vi "get object tags.vi"(1 "can select all services":bool, 2 "Object":string, 5 "error in (no error)":errorcluster) -> (16 "services":string[](array[string]), 17 "descriptors":string[](array[string]), 19 "error out":errorcluster)   [LabVIEW 2014, in "PTUtils.lvlib"]
doc: "Gets the services published by an object by queying its DIM server."
uses:
  PTUtils.lvlib
  CSCore/CSSystem/CoreLib/CoreLib.lvlib
  CSlibraries/UtilityLib/UtilityLib.lvlib
  CSlibraries-extern/DimLVEvent/LVDimInterface/LVDimInterface.lvlib
  CSCore/CSSystem/CSSystemLib/CSSystemLib.lvlib
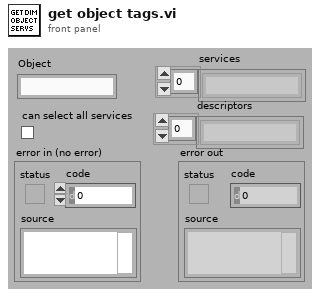
[diagram p1: front panel]
types:
  T1 = cluster{"string without white spaces":string, "string without white spaces":string}
  T2 = cluster{"string without white spaces":string, "string without white spaces":string}[]
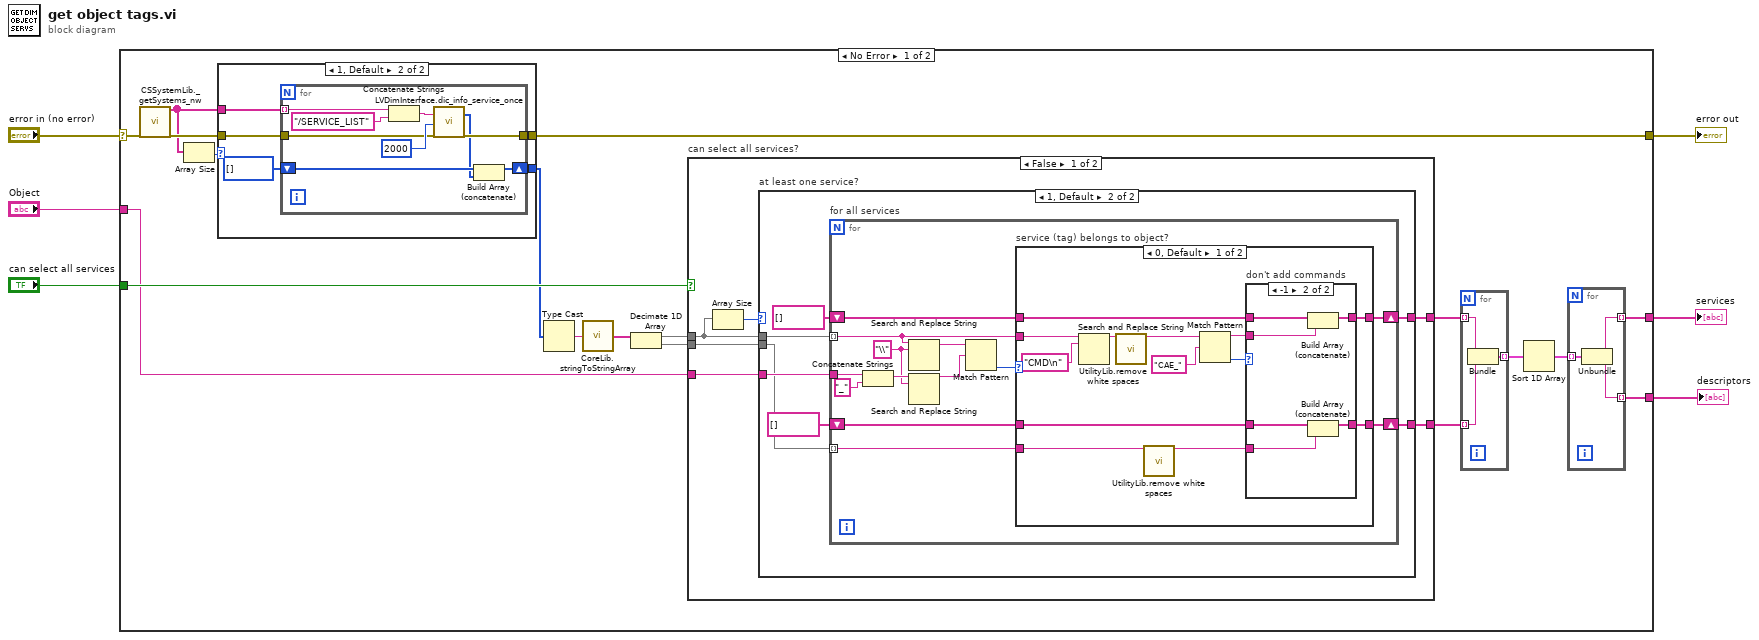
[diagram p0: block diagram]
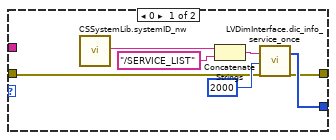
[diagram p2: hidden frame]
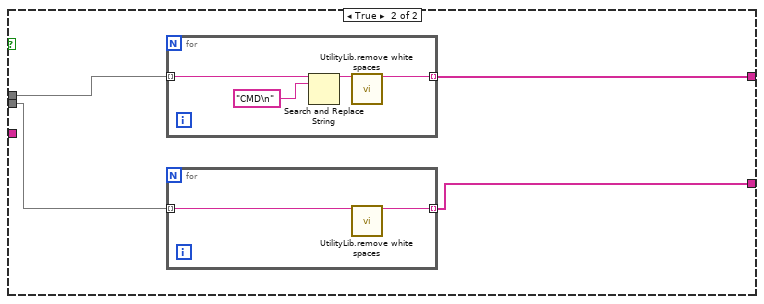
[diagram p6: hidden frame]
diagram:
  n1 = case shown="No Error" "error in (no error)" {
    selector: "error in (no error)" -> [w17 w111]
    tunnel: [w23 w111] -> w6
    tunnel: "can select all services" -> [w24 _]
    tunnel: "Object" -> [w14 _]
    tunnel: [w8 _] -> w2
    tunnel: [w7 _] -> w1
    frame No Error {
      n2 = call "CSSystemLib._getSystems_nw.vi"("error in (no error)"=w17) -> ("CSSystems"=w16:string[], "error out"=w18:errorcluster)  [unwired: 16 in, 1 out]
      n3 = Array Size(array=w16) -> (size(s)=w15:i32)
      n4 = case shown="1, Default" w15 {
        tunnel: [w32 w42] -> w23
        tunnel: [w34 w41] -> w22
        tunnel: w18 -> [w31 w39]
        tunnel: w16 -> [_ w38]
        frame 0 {
          n5 = call "CSSystemLib.systemID_nw.vi"() -> ("systemID out"=w33:string)  [unwired: 18 in, 1 out]
          n6 = Concatenate Strings(w33, "/SERVICE_LIST" ("string")) -> (w36:string)
          n7 = call "LVDimInterface.dic_info_service_once.vi"("serviceName"=w36, "timeout [ms]"=u32 2000, "error in (no error)"=w31) -> ("data"=w34:i8[], "error out"=w32:errorcluster)  [unwired: 13 in, 2 out]
        }
        frame 1, Default {
          n8 = for {
            tunnel: [w51] -> w42
            shift-right: [w45] -> w41
            shift-left: i8[] [] ("data") -> [w47]
            tunnel: w38 -> [w48] mode=indexing
            tunnel: w39 -> [w44]
            n9 = Concatenate Strings(w48, "/SERVICE_LIST" ("string")) -> (w50:string)
            n10 = call "LVDimInterface.dic_info_service_once.vi"("serviceName"=w50, "timeout [ms]"=u32 2000, "error in (no error)"=w44) -> ("data"=w46:i8[], "error out"=w51:errorcluster)  [unwired: 13 in, 2 out]
            n11 = Build Array (concatenate)(w47, w46) -> (w45:i8[])
          }
        }
      }
      n12 = Type Cast(x=w22) -> (*(type *) &x=w19:string)  [unwired: 1 in]
      n13 = call "CoreLib.stringToStringArray.vi"("String"=w19) -> ("Array"=w21:string[])
      n14 = Decimate 1D Array(w21) -> (w20:string[], w13:string[])
      n15 = case "can select all services?" shown="False" w24 {
        tunnel: [w56 w103] -> w11
        tunnel: w20 -> [w54 w104]
        tunnel: w14 -> [w55 _]
        tunnel: w13 -> [w53 w102]
        tunnel: [w52 w101] -> w10
        frame False {
          n16 = Array Size(array=w54) -> (size(s)=w57:i32)
          n17 = case "at least one service?" shown="1, Default" w57 {
            tunnel: [_ w63] -> w56
            tunnel: w54 -> [_ w62]
            tunnel: w55 -> [_ w61]
            tunnel: w53 -> [_ w60]
            tunnel: [_ w58] -> w52
            frame 0 {
            }
            frame 1, Default {
              n18 = for "for all services" {
                shift-right: [w74] -> w63
                shift-left: string[] [] -> [w75]
                tunnel: w62 -> [w70] mode=indexing
                tunnel: w61 -> [w77]
                tunnel: w60 -> [w67] mode=indexing
                shift-right: [w65] -> w58
                shift-left: string[] [] -> [w66]
                w68 = "\\" ("search string")
                n19 = Concatenate Strings(w77, "_" ("string")) -> (w72:string)
                n20 = Search and Replace String(input string=w70, search string=w68) -> (result string=w69:string)  [unwired: 6 in, 3 out]
                n21 = Search and Replace String(input string=w72, search string=w68) -> (result string=w71:string)  [unwired: 6 in, 3 out]
                n22 = Match Pattern(string=w69, regular expression=w71) -> (offset past match=w73:i32)  [unwired: 1 in, 3 out]
                n23 = case "service (tag) belongs to object?" shown="0, Default" w73 {
                  tunnel: [w89 w100] -> w74
                  tunnel: w75 -> [w90 w100]
                  tunnel: w70 -> [w88 _]
                  tunnel: w67 -> [w81 _]
                  tunnel: w66 -> [w80 w99]
                  tunnel: [w79 w99] -> w65
                  frame 0, Default {
                    n24 = Search and Replace String(input string=w88, search string="CMD\n" ("substring (\"\")")) -> (result string=w86:string)  [unwired: 6 in, 3 out]
                    n25 = call "UtilityLib.remove white spaces.vi"("string with blanks"=w86) -> ("string without white spaces"=w85:string)  [unwired: 14 in, 4 out]
                    n26 = call "UtilityLib.remove white spaces.vi"("string with blanks"=w81) -> ("string without white spaces"=w78:string)  [unwired: 14 in, 4 out]
                    n27 = Match Pattern(string=w85, regular expression="CAE_") -> (before substring=w82:string, offset past match=w83:i32)  [unwired: 1 in, 2 out]
                    n28 = case "don't add commands" shown="-1" w83 {
                      tunnel: w90 -> [w92 w98]
                      tunnel: [w92 w97] -> w89
                      tunnel: w82 -> [_ w96]
                      tunnel: w80 -> [w91 w95]
                      tunnel: [w91 w94] -> w79
                      tunnel: w78 -> [_ w93]
                      frame 0, Default {
                      }
                      frame -1 {
                        n29 = Build Array (concatenate)(w98, w96) -> (w97:string[])
                        n30 = Build Array (concatenate)(w95, w93) -> (w94:string[])
                      }
                    }
                  }
                  frame -1 {
                  }
                }
              }
            }
          }
        }
        frame True {
          n31 = for {
            tunnel: w104 -> [w108] mode=indexing
            tunnel: [w107] -> w103 mode=indexing
            n32 = Search and Replace String(input string=w108, search string="CMD\n" ("substring (\"\")")) -> (result string=w109:string)  [unwired: 6 in, 3 out]
            n33 = call "UtilityLib.remove white spaces.vi"("string with blanks"=w109) -> ("string without white spaces"=w107:string)  [unwired: 14 in, 4 out]
          }
          n34 = for {
            tunnel: [w106] -> w101 mode=indexing
            tunnel: w102 -> [w105] mode=indexing
            n35 = call "UtilityLib.remove white spaces.vi"("string with blanks"=w105) -> ("string without white spaces"=w106:string)  [unwired: 14 in, 4 out]
          }
        }
      }
      n36 = for {
        tunnel: w11 -> [w30] mode=indexing
        tunnel: [w29] -> w9 mode=indexing
        tunnel: w10 -> [w28] mode=indexing
        n37 = Bundle("string without white spaces"=w30, "string without white spaces"=w28) -> (w29:T1)  [unwired: 1 in]
      }
      n38 = Sort 1D Array(array=w9) -> (sorted array=w12:T2)
      n39 = for {
        tunnel: w12 -> [w25] mode=indexing
        tunnel: [w27] -> w8 mode=indexing
        tunnel: [w26] -> w7 mode=indexing
        n40 = Unbundle(w25) -> ("string without white spaces"=w27:string, "string without white spaces"=w26:string)
      }
    }
    frame Error {
    }
  }
  "error out" <- w6
  "services" <- w2
  "descriptors" <- w1
